vi "Write Server Hostname.vi"(8 "error in (no error)":errorcluster, 10 "Server Hostname":string, 11 "SSL Client Socket in":refnum<class "SSL Client Socket.lvclass">) -> (0 "error out":errorcluster, 3 "SSL Client Socket out":refnum<class "SSL Client Socket.lvclass">)   [LabVIEW 2013, in "OpenSSL Socket.lvlib" / "SSL Client Socket.lvclass"]
uses:
  SSL Client Socket.lvclass
  SSL Client Socket.lvclass/SSL Client Socket.ctl
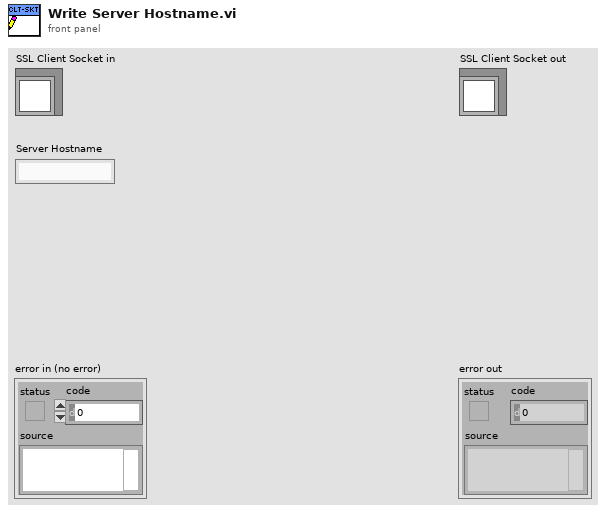
[diagram p1: front panel]
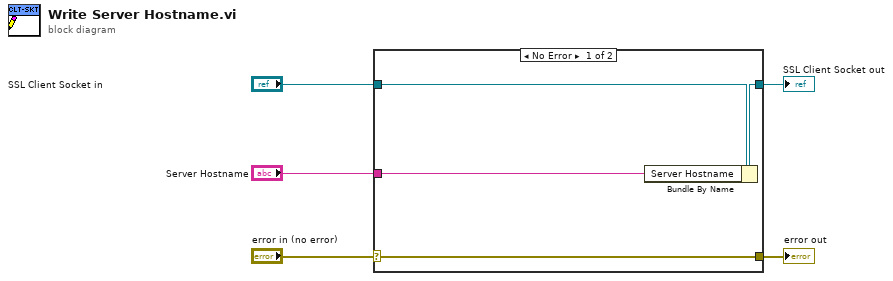
[diagram p0: block diagram]
diagram:
  n1 = case shown="No Error" "error in (no error)" {
    selector: "error in (no error)" -> [w9 w10]
    tunnel: [w9 w10] -> w4
    tunnel: [w7 w11] -> w2
    tunnel: "SSL Client Socket in" -> [w8 w11]
    tunnel: "Server Hostname" -> [w6 _]
    frame No Error {
      n2 = Bundle By Name(cluster=w8, "Server Hostname"=w6) -> (w7:refnum<class "SSL Client Socket.lvclass">)
    }
    frame Error {
    }
  }
  "error out" <- w4
  "SSL Client Socket out" <- w2
